vi "M9003Reset.vi"(0 "HANDLE":i32) -> ()   [LabVIEW 2009]
uses:
  M9003api.dll
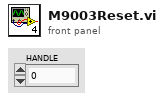
[diagram p1: front panel]
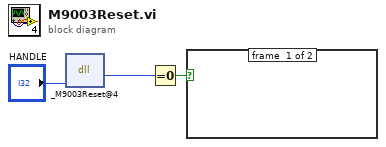
[diagram p0: block diagram]
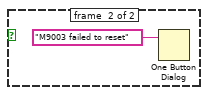
[diagram p2: hidden frame]
diagram:
  n1 = dll-call lib="H:/Mover_2009/Sub_Vis/M9003Commands/M9003api.dll" fn="_M9003Reset@4" label="M9003Reset"("Handle"="HANDLE") -> ("return type"=w2:i32)  [unwired: 4 in, 2 out]
  n2 = Equal To 0?(x=w2) -> (x = 0?=w1:bool)
  n3 = case shown="True" w1 {
    frame #0 {
    }
    frame #1 {
      n4 = One Button Dialog(message="M9003 failed to reset") -> ()  [unwired: 1 in, 1 out]
    }
  }
